vi "Autonomous Independent.vi"() -> ()   [LabVIEW 2013]
doc: "This VI is called when autonomous begins, and will automatically be terminated when autonomous ends. You can carry out timed or sensor driven robot movement independently without needing to return to the caller."
uses:
  Robot Global Data.vi
  <vilib>/Rock Robotics/WPI/RobotDrive/WPI_RobotDriveGetSetRefNum.vi
  <vilib>/Rock Robotics/WPI/RobotDrive/WPI_RobotDriveArcadeDrive_Standard(NoSaturation).vi
  <vilib>/Rock Robotics/WPI/Joystick/WPI_JoystickGetSetRefNum.vi
panel:
  out "Current Movement, for debugging":T1 {"Y Joystick Value" scale=1.0..-1.0; "X Joystick Value" scale=-1.0..1.0}
  in  "Array of robot movements":T2(array[cluster]) {"Y Joystick Value" scale=1.0..-1.0; "X Joystick Value" scale=-1.0..1.0}
  # "Be sure to right-click and choose Data Operations>>Make Current Value default if you want to save the array values with the VI"
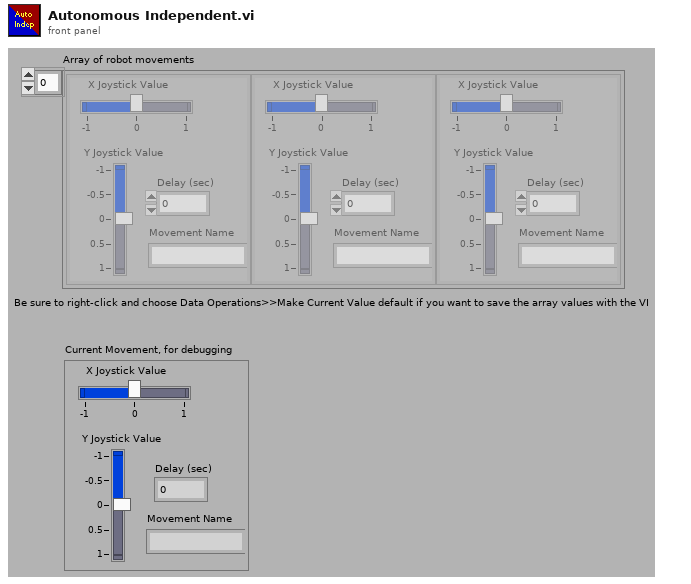
[diagram p1: front panel]
types:
  T1 = cluster{"X Joystick Value":dbl, "Y Joystick Value":dbl, "Delay (sec)":dbl, "Movement Name":string}
  T2 = cluster{"X Joystick Value":dbl, "Y Joystick Value":dbl, "Delay (sec)":dbl, "Movement Name":string}[]
  T3 = typedef "WPI_JoystickDevRef.ctl" = cluster{"Device":T4}
  T4 = typedef "WPI_JoystickDeviceEnum.ctl" = enum16{"USB 1", "USB 2", "USB 3", "USB 4", "Kinect 1", "Kinect 2"}
  T5 = cluster{"axis 1 (x)":dbl, "axis 2 (y)":dbl, "axis 3 (throttle)":dbl, "axis 4":dbl, "axis 5":dbl, "axis 6":dbl}
  T6 = typedef "WPI_RobotDriveDevRef.ctl" = cluster{"DevStatus":errorcluster, "Motors[]":T7[], "Square Inputs":bool, "Max Output":dbl, "Isochronous":bool}
  T7 = typedef "WPI_MotorControlDeviceRef.ctl" = cluster{"DeviceStatus":errorcluster, "Type":enum16{"PWM", "CAN"}, "PWM":cluster{"Digital Module":T8, "PWM Channel":T9, "DeadBand":T10}, "CAN":cluster{"Device Number":u8, "Control Mode":T11, "Semaphore":T12, "Max Vout":dbl}, "Invert":bool, "TransformRef":T13, "InvTransformRef":T13}
  T8 = typedef "FPGA_TypedefDigitalModule.ctl" = enum16{"Digital Module 1", "Digital Module 2"}
  T9 = typedef "FPGA_DIOPWMChannel.ctl" = enum8{"PWM 1", "PWM 2", "PWM 3", "PWM 4", "PWM 5", "PWM 6", "PWM 7", "PWM 8", "PWM 9", "PWM 10", "Invalid"}
  T10 = typedef "WPI_PWMDeadband.ctl" = cluster{"Name":string, "maxPositivePwm":i32, "minPositivePwm":i32, "centerPwm":i32, "maxNegativePwm":i32, "minNegativePwm":i32, "angularRange":u16}
  T11 = typedef "WPI_CANJaguar_ControlMode.ctl" = enum8{"Percent VBus", "Current", "Speed", "Position", "Voltage"}
  T12 = typedef "Semaphore RefNum" = refnum<k1>
  T13 = typedef "WPI_PWMTransform_ConPane.ctl" = refnum<vi>
  T14 = typedef "WPI_DigitalInputDevRef.ctl" = cluster{"DevStatus":errorcluster, "DIO Channel":T15, "Digital Module":T8}
  T15 = typedef "FPGA_DIOChannel.ctl" = enum8{"DIO 1", "DIO 2", "DIO 3", "DIO 4", "DIO 5", "DIO 6", "DIO 7", "DIO 8", "DIO 9", "DIO 10", "DIO 11", "DIO 12", "DIO 13", "DIO 14", "Invalid"}
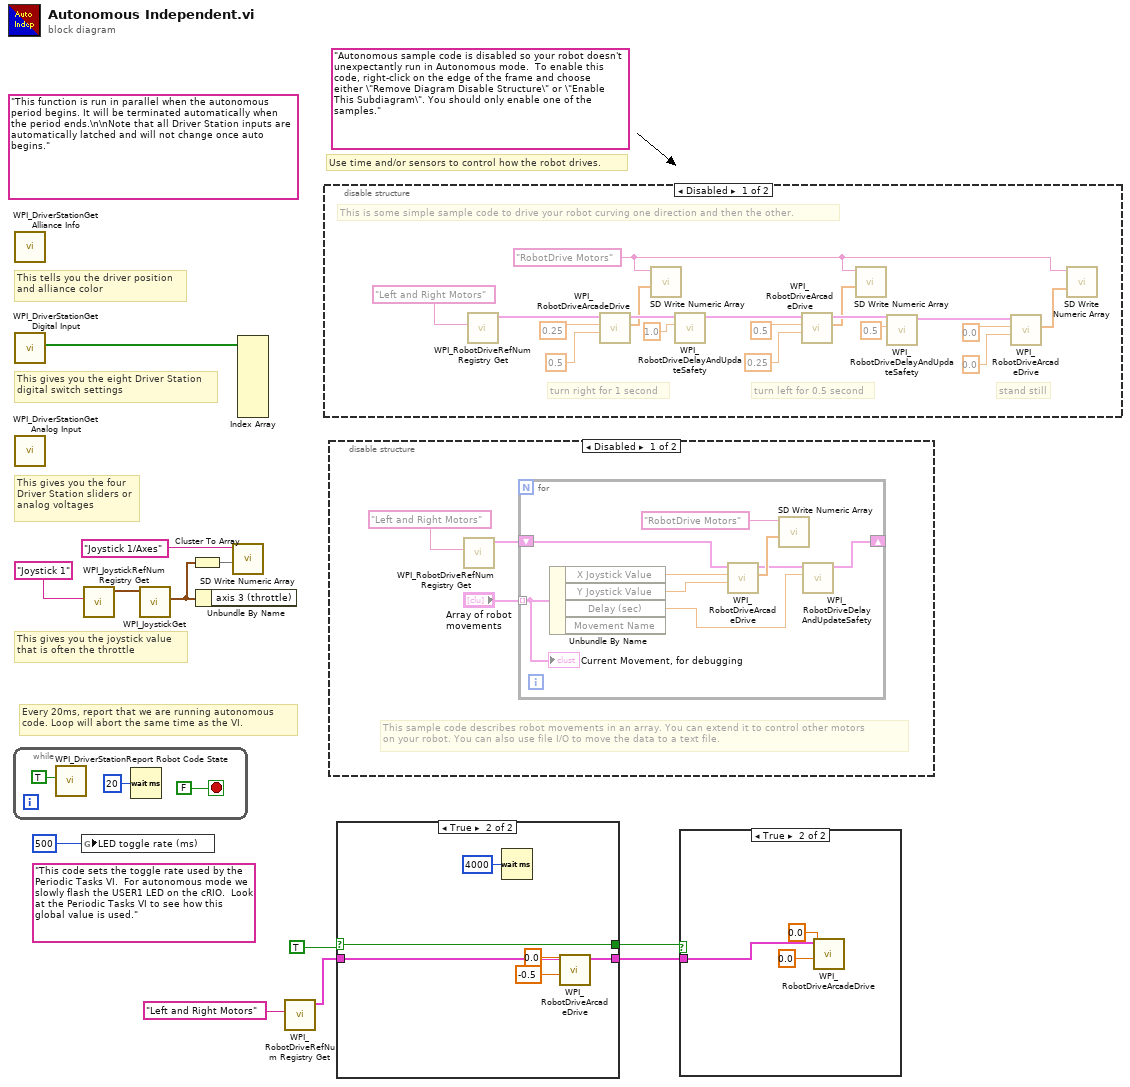
[diagram p0: block diagram]
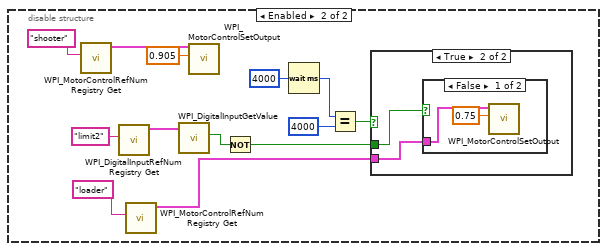
[diagram p5: hidden frame]
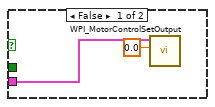
[diagram p6: hidden frame]
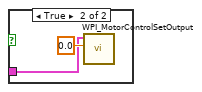
[diagram p7: hidden frame]
diagram:
  (unwired) "This code sets the toggle rate used by the Periodic Tasks VI.  For autonomous mode we slowly flash the USER1 LED on the cRIO.  Look at the Periodic Tasks VI to see how this global value is used."
  (unwired) "Autonomous sample code is disabled so your robot doesn't unexpectantly run in Autonomous mode.  To enable this code, right-click on the edge of the frame and choose either \"Remove Diagram Disable Structure\" or \"Enable This Subdiagram\". You should only enable one of the samples."
  (unwired) "This function is run in parallel when the autonomous period begins. It will be terminated automatically when the period ends.\n\nNote that all Driver Station inputs are automatically latched and will not change once auto begins."
  # "Every 20ms, report that we are running autonomous\ncode. Loop will abort the same time as the VI."
  # "This gives you the joystick value\nthat is often the throttle"
  # "Use time and/or sensors to control how the robot drives."
  # "This tells you the driver position\nand alliance color"
  # "This gives you the eight Driver Station\ndigital switch settings"
  # "This gives you the four\nDriver Station sliders or\nanalog voltages"
  n1 = while {
    stop <- FALSE stop-if-true
    n2 = call <vilib>:"WPI_DriverStationReport Robot Code State.vi"("Autonomous"=TRUE) -> ()  [unwired: 10 in, 1 out]
    n3 = Wait (ms)(milliseconds to wait=u32 20) -> ()  [unwired: 1 out]
  }
  n4 = call <vilib>:"WPI_DriverStationGet Alliance Info.vi"() -> ()  [unwired: 12 out]
  n5 = call <vilib>:"WPI_DriverStationGet Digital Input.vi"() -> ("Driver Station Digital Input (1-8)"=w12:bool[])  [unwired: 11 out]
  n6 = call <vilib>:"WPI_DriverStationGet Analog Input.vi"() -> ()  [unwired: 12 out]
  n7 = global write "Robot Global Data.vi" "LED toggle rate (ms)"(u32 500 ("LED ms toggle rate")) -> ()
  n8 = call <vilib>:"WPI_JoystickRefNum Registry Get.vi"("refnum name"="Joystick 1") -> ("JoystickDevRef"=w10:T3)  [unwired: 1 in, 9 out]
  n9 = call <vilib>:"WPI_JoystickGet.vi"("JoystickDevRef"=w10) -> ("Axes"=w7:T5)  [unwired: 1 in, 5 out]
  n10 = Cluster To Array(cluster=w7) -> (array=w8:dbl[])
  n11 = Unbundle By Name(w7) -> ()  [unwired: 1 out]
  n12 = call <vilib>:"SD Write Numeric Array.vi"("Numeric Array"=w8, "Name"="Joystick 1/Axes") -> ()  [unwired: 8 in, 2 out]
  n13 = Index Array(array=w12) -> ()  [unwired: 8 in, 8 out]
  n14 = call <vilib>:"WPI_RobotDriveRefNum Registry Get.vi"("refnum name"="Left and Right Motors") -> ("RobotDriveDevRef"=w1:T6)  [unwired: 1 in, 9 out]
  n15 = disable-structure shown="Disabled" {
    frame Disabled {
      w16 = "RobotDrive Motors" ("Name")
      # "This is some simple sample code to drive your robot curving one direction and then the other."
      # "stand still"
      # "turn left for 0.5 second"
      # "turn right for 1 second"
      n16 = call <vilib>:"WPI_RobotDriveRefNum Registry Get.vi"("refnum name"="Left and Right Motors") -> ("RobotDriveDevRef"=w20:T6)  [unwired: 1 in, 9 out]
      n17 = call-poly <vilib>:"WPI_RobotDriveArcadeDrive.vi"("Y axis value"=0.5 ("X axis value"), "X axis value"=0.25, "RobotDriveDevRef"=w20) -> ("Motor Values"=w19:dbl[], "RobotDriveDevRef"=w27:T6)  [unwired: 1 in, 6 out]
      n18 = call <vilib>:"SD Write Numeric Array.vi"("Numeric Array"=w19, "Name"=w16) -> ()  [unwired: 8 in, 2 out]
      n19 = call <vilib>:"WPI_RobotDriveDelayAndUpdateSafety.vi"("Delay (s)"=1.0, "RobotDriveDevRef"=w27) -> ("RobotDriveDevRef 2"=w26:T6)  [unwired: 8 in, 1 out]
      n20 = call-poly <vilib>:"WPI_RobotDriveArcadeDrive.vi"("Y axis value"=0.25 ("X axis value"), "X axis value"=0.5, "RobotDriveDevRef"=w26) -> ("Motor Values"=w18:dbl[], "RobotDriveDevRef"=w25:T6)  [unwired: 1 in, 6 out]
      n21 = call <vilib>:"SD Write Numeric Array.vi"("Numeric Array"=w18, "Name"=w16) -> ()  [unwired: 8 in, 2 out]
      n22 = call <vilib>:"WPI_RobotDriveDelayAndUpdateSafety.vi"("Delay (s)"=0.5, "RobotDriveDevRef"=w25) -> ("RobotDriveDevRef 2"=w24:T6)  [unwired: 8 in, 1 out]
      n23 = call-poly <vilib>:"WPI_RobotDriveArcadeDrive.vi"("Y axis value"=0.0 ("X axis value"), "X axis value"=0.0, "RobotDriveDevRef"=w24) -> ("Motor Values"=w17:dbl[])  [unwired: 1 in, 7 out]
      n24 = call <vilib>:"SD Write Numeric Array.vi"("Numeric Array"=w17, "Name"=w16) -> ()  [unwired: 8 in, 2 out]
    }
    frame Enabled {
      n25 = call <vilib>:"WPI_MotorControlRefNum Registry Get.vi"("refnum name"="shooter") -> ("MotorControlDevRef"=w46:T7)  [unwired: 9 in, 1 out]
      n26 = call <vilib>:"WPI_DigitalInputRefNum Registry Get.vi"("refnum name"="limit2") -> ("DigitalInputDevRef"=w41:T14)  [unwired: 9 in, 1 out]
      n27 = call <vilib>:"WPI_MotorControlRefNum Registry Get.vi"("refnum name"="loader") -> ("MotorControlDevRef"=w35:T7)  [unwired: 9 in, 1 out]
      n28 = call <vilib>:"WPI_DigitalInputGetValue.vi"("DigitalInputDevRef"=w41) -> ("Value"=w42:bool)  [unwired: 8 in, 2 out]
      n29 = call <vilib>:"WPI_MotorControlSetOutput.vi"("Output"=0.905, "MotorControlDevRef"=w46) -> ()  [unwired: 7 in, 3 out]
      n30 = Not(x=w42) -> (.not. x?=w34:bool)
      n31 = Wait (ms)(milliseconds to wait=u32 4000) -> (millisecond timer value=w38:u32)
      n32 = Equal?(x=w38, y=u32 4000) -> (x = y?=w39:bool)
      n33 = case shown="True" w39 {
        tunnel: w35 -> [w48 w50]
        tunnel: w34 -> [_ w49]
        frame False {
          n34 = call <vilib>:"WPI_MotorControlSetOutput.vi"("Output"=0.0, "MotorControlDevRef"=w48) -> ()  [unwired: 7 in, 3 out]
        }
        frame True {
          n35 = case shown="False" w49 {
            tunnel: w50 -> [w52 w53]
            frame False {
              n36 = call <vilib>:"WPI_MotorControlSetOutput.vi"("Output"=0.75, "MotorControlDevRef"=w52) -> ()  [unwired: 7 in, 3 out]
            }
            frame True {
              n37 = call <vilib>:"WPI_MotorControlSetOutput.vi"("Output"=0.0, "MotorControlDevRef"=w53) -> ()  [unwired: 7 in, 3 out]
            }
          }
        }
      }
    }
  }
  n38 = disable-structure shown="Disabled" {
    frame Disabled {
      # "This sample code describes robot movements in an array. You can extend it to control other motors\non your robot. You can also use file I/O to move the data to a text file."
      n39 = call <vilib>:"WPI_RobotDriveRefNum Registry Get.vi"("refnum name"="Left and Right Motors") -> ("RobotDriveDevRef"=w56:T6)  [unwired: 1 in, 9 out]
      n40 = for {
        shift-right: [w62] -> _
        shift-left: w56 -> [w63]
        tunnel: "Array of robot movements" -> [w58] mode=indexing
        n41 = Unbundle By Name(w58) -> ("X Joystick Value"=w61:dbl, "Y Joystick Value"=w60:dbl, "Delay (sec)"=w59:dbl)  [unwired: 1 out]
        n42 = call-poly <vilib>:"WPI_RobotDriveArcadeDrive.vi"("Y axis value"=w60, "X axis value"=w61, "RobotDriveDevRef"=w63) -> ("Motor Values"=w65:dbl[], "RobotDriveDevRef"=w64:T6)  [unwired: 1 in, 6 out]
        n43 = call <vilib>:"SD Write Numeric Array.vi"("Numeric Array"=w65, "Name"="RobotDrive Motors") -> ()  [unwired: 8 in, 2 out]
        n44 = call <vilib>:"WPI_RobotDriveDelayAndUpdateSafety.vi"("Delay (s)"=w59, "RobotDriveDevRef"=w64) -> ("RobotDriveDevRef 2"=w62:T6)  [unwired: 8 in, 1 out]
        "Current Movement, for debugging" <- w58
      }
    }
    frame Enabled {
    }
  }
  n45 = case shown="True" TRUE {
    selector: TRUE -> [w68 w73]
    tunnel: [w68 w73] -> w4
    tunnel: [w67 w70] -> w3
    tunnel: w1 -> [w67 w69]
    frame False {
    }
    frame True {
      n46 = Wait (ms)(milliseconds to wait=u32 4000) -> ()  [unwired: 1 out]
      n47 = call-poly <vilib>:"WPI_RobotDriveArcadeDrive.vi"("Y axis value"=-0.5, "X axis value"=0.0, "RobotDriveDevRef"=w69) -> ("RobotDriveDevRef"=w70:T6)  [unwired: 6 in, 2 out]
    }
  }
  n48 = case shown="True" w4 {
    tunnel: w3 -> [_ w77]
    frame False {
    }
    frame True {
      n49 = call-poly <vilib>:"WPI_RobotDriveArcadeDrive.vi"("Y axis value"=0.0, "X axis value"=0.0, "RobotDriveDevRef"=w77) -> ()  [unwired: 6 in, 3 out]
    }
  }
